vi "PLS Main.vi"(8 "error in (no error)":errorcluster, 9 "Aufnahme":bool caption="Record", 10 "Stop":bool, 11 "Play":bool) -> (0 "error out":errorcluster, 3 "Set Information":T1 {"Channels"."Intensität" min=0.0 max=100.0 step=1.0 format="%#.0f"})   [LabVIEW 2010]
doc: "User Interface für die Party Licht Steuerung"
uses:
  Controls/tlc_Cue_Information.ctl
  Controls/channel.ctl
  Controls/tlc_Consumer Control.ctl
  Controls/tlc_Functions.ctl
  Controls/tlc_User Interface Command.ctl
  Controls/tlc_User Interface Data Type.ctl
  Modules/Error/tlc_Error Module Command Control.ctl
  Modules/File/tlc_File_Command Control.ctl
  Modules/Cue/tlc_Cue_Information Command.ctl
  Integration/tlc_Record.vi
  Integration/tlc_Record Dialog Box.vi
panel:
  out "Cue List":i32(listbox)
  # "Ablaufkontrolle"
  # "Set Information"
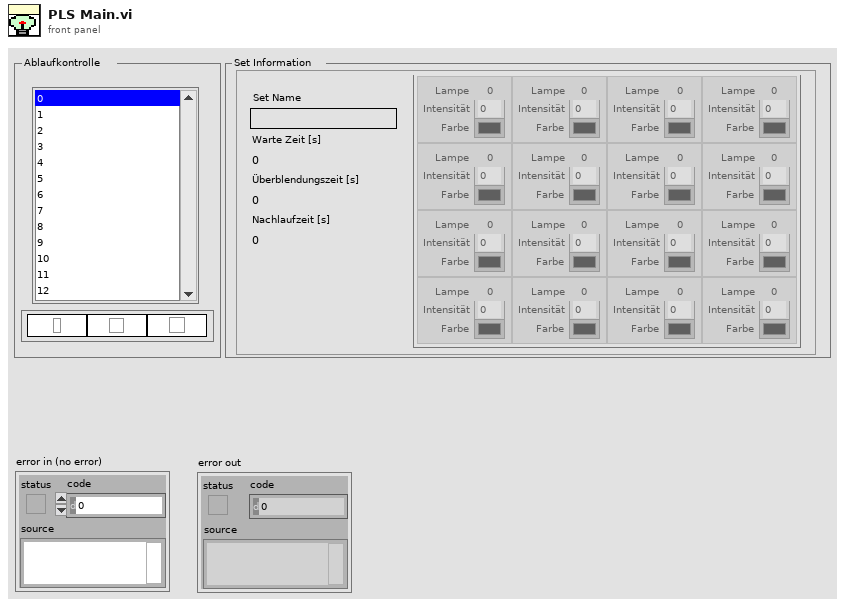
[diagram p1: front panel]
types:
  T1 = typedef "tlc_Cue_Information.ctl" = cluster{"Cue Name":string, "Wait Time (s)":u32, "Fade Time (s)":u32, "Follow Time (s)":u32, "Channels":T2[][]}
  T2 = typedef "channel.ctl" = cluster{"Intensität":dbl, " Farbe":u32, "Channel":i32}
  T3 = typedef "tlc_Error Module Command Control.ctl" = enum16{"Initialize", "Handle Errors", "Report Errors"}
  T4 = typedef "tlc_User Interface Command.ctl" = cluster{"Data Type":T5, "Data":variant}
  T5 = typedef "tlc_User Interface Data Type.ctl" = enum16{"Initialize", "Initialize Front Panel", "Update Front Panel Channels", "Select Cue in Cue List", "Enable/Disable Front Panel Controls", "Update Cue List", "Stop"}
  T6 = typedef "tlc_Consumer Control.ctl" = cluster{"Command":T7, "Data":variant}
  T7 = typedef "tlc_Functions.ctl" = enum16{"Initialize", "Record", "Load", "Save", "Play", "Stop", "Exit"}
  T8 = typedef "tlc_File_Command Control.ctl" = enum16{"Init", "Speicher Lichtersets", "Lade Lichtersets", "Ende"}
  T9 = typedef "tlc_Cue_Information Command.ctl" = enum16{"Add Lichtset", "Get Lichtset Werte", "Set Lichtset Werte", "Get Anzahl Lichtersets", "Init", "Get Leeres Lichterset"}
  T10 = enum32{"invalid app kind", "Development System", "Run Time System", "Student Edition", "Embedded LabVIEW", "Evaluation", "Custom"}
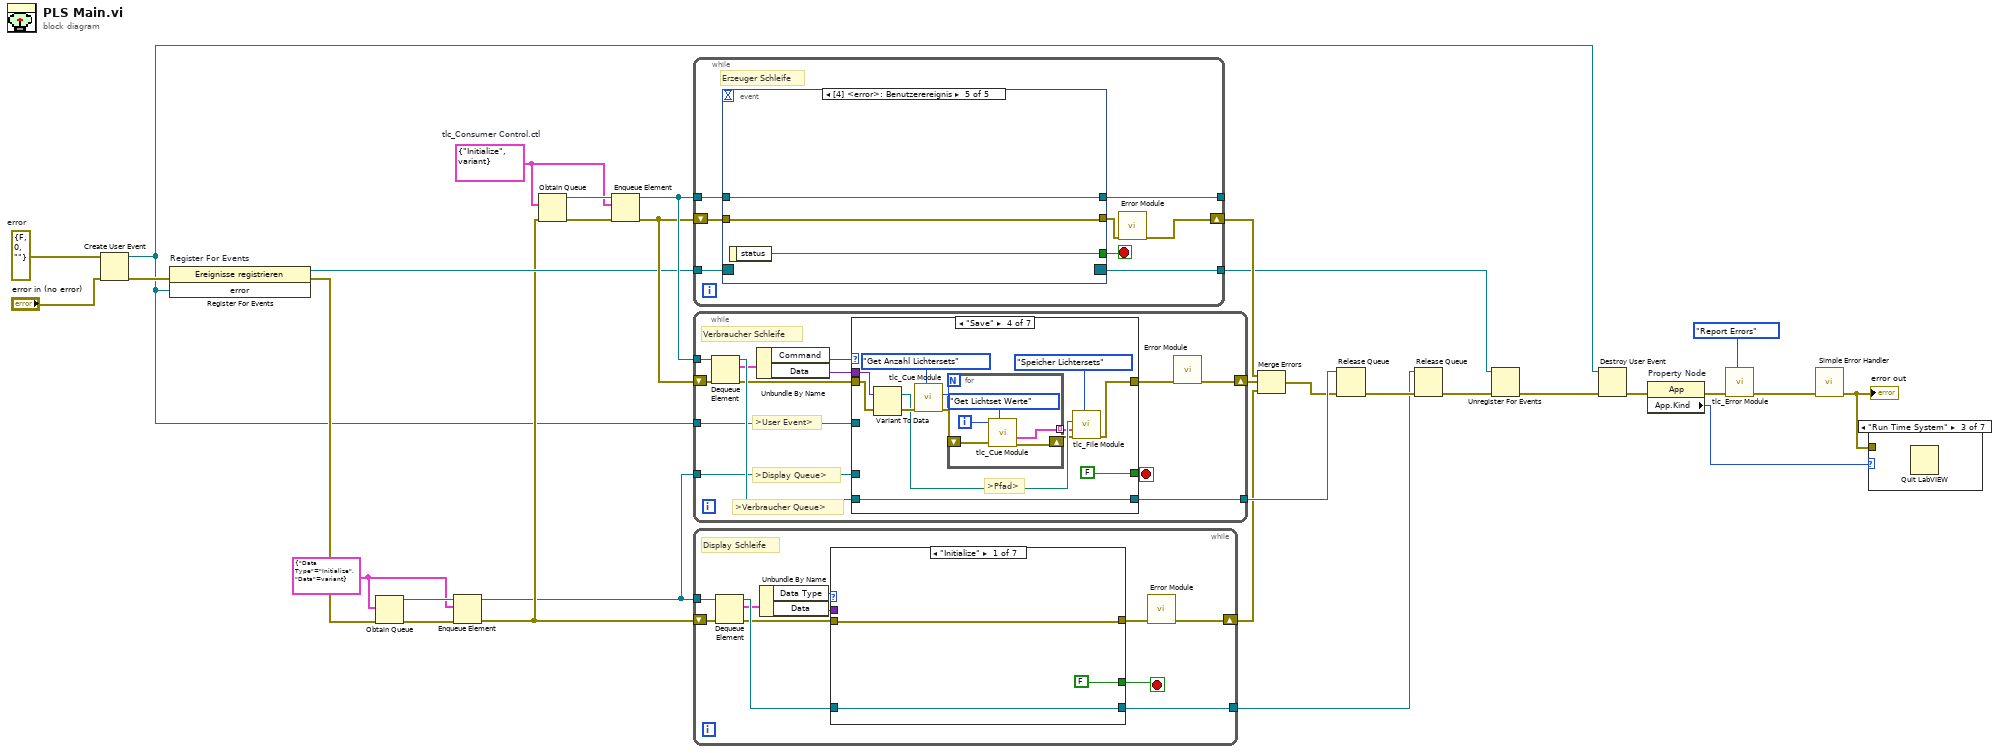
[diagram p0: block diagram]
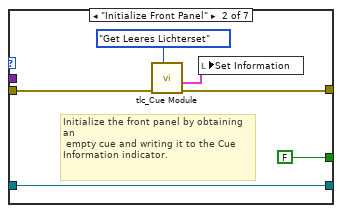
[diagram p8: hidden frame]
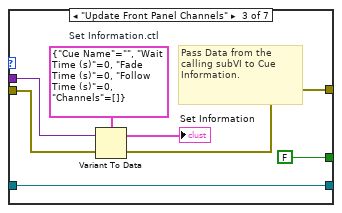
[diagram p9: hidden frame]
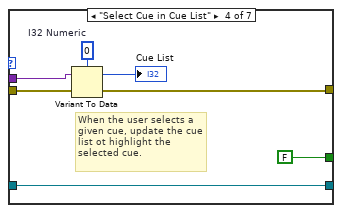
[diagram p10: hidden frame]
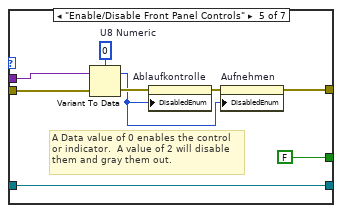
[diagram p11: hidden frame]
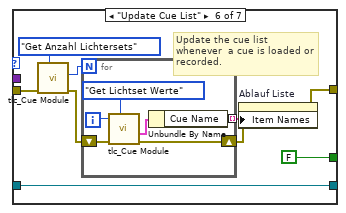
[diagram p12: hidden frame]
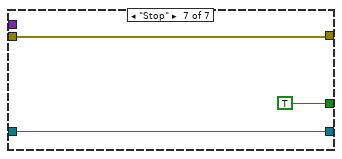
[diagram p13: hidden frame]
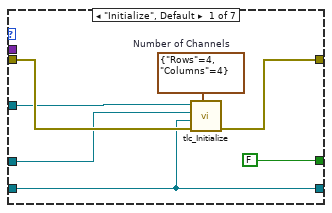
[diagram p14: hidden frame]
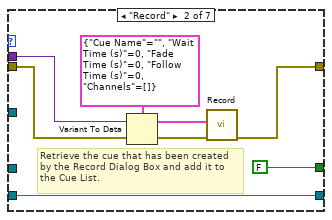
[diagram p15: hidden frame]
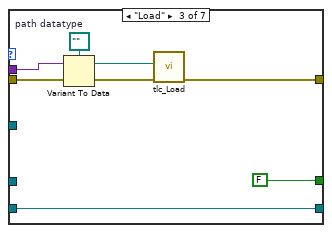
[diagram p16: hidden frame]
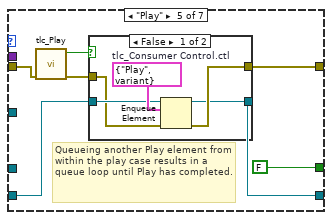
[diagram p17: hidden frame]
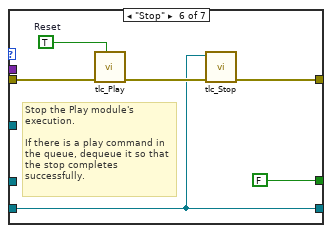
[diagram p19: hidden frame]
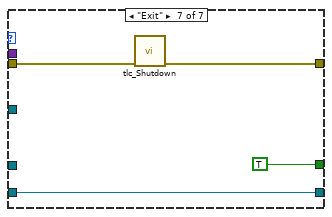
[diagram p20: hidden frame]
diagram:
  w15 = T4 {"Data Type"=enum."Initialize", "Data"=variant} ("tlc_User Interface Command.ctl")
  w27 = errorcluster {"status"=FALSE, "code"=0, "source"=""}  # error
  w29 = T6 {"Command"=enum."Initialize", "Data"=variant}  # tlc_Consumer Control.ctl
  n1 = Create User Event(user event datatype=w27, error in="error in (no error)") -> (user event=w9:refnum<user-event>, error out=w26:errorcluster)
  n2 = register-events "Register For Events"(error in=w26, w9) -> (reference out=w25:refnum<event-registration>, error out=w14:errorcluster)  [unwired: 1 in]
  n3 = Obtain Queue(element data type=w15, error in (no error)=w14) -> (queue out=w16:refnum<queue>, error out=w17:errorcluster)  [unwired: 3 in, 1 out]
  n4 = Enqueue Element(queue=w16, element=w15, error in (no error)=w17) -> (queue out=w8:refnum<queue>, error out=w13:errorcluster)  [unwired: 1 in, 1 out]
  n5 = Obtain Queue(element data type=w29, error in (no error)=w13) -> (queue out=w32:refnum<queue>, error out=w31:errorcluster)  [unwired: 3 in, 1 out]
  n6 = Enqueue Element(queue=w32, element=w29, error in (no error)=w31) -> (queue out=w30:refnum<queue>, error out=w28:errorcluster)  [unwired: 1 in, 1 out]
  n7 = while {
    shift-right: [w33] -> w23
    shift-left: w28 -> [w42]
    tunnel: w30 -> [w45]
    tunnel: [w43] -> w21
    tunnel: w9 -> [w37]
    tunnel: w8 -> [w36]
    stop <- w38 stop-if-true
    # ">Display Queue>"
    # ">Verbraucher Queue>"
    # ">User Event>"
    # "Verbraucher Schleife"
    n8 = Dequeue Element(queue=w45, error in (no error)=w42) -> (queue out=w44:refnum<queue>, element=w41:T6, error out=w39:errorcluster)  [unwired: 1 in, 1 out]
    n9 = Unbundle By Name(w41) -> ("Command"=w40:T7, "Data"=w35:variant)
    n10 = case shown="\"Save\"" w40 {
      tunnel: w44 -> [w48 w60 w68 w81 w89 w101 w110]
      tunnel: [w48 w60 w68 w81 w87 w101 w110] -> w43
      tunnel: w39 -> [w50 w53 w65 w78 w92 w104 w108]
      tunnel: [w49 w57 w62 w70 w88 w103 w107] -> w34
      tunnel: [FALSE FALSE FALSE FALSE FALSE FALSE TRUE] -> w38
      tunnel: w35 -> [_ w54 w66 w79 _ _ _]
      tunnel: w37 -> [w47 _ _ _ _ _ _]
      tunnel: w36 -> [w46 _ _ _ _ _ _]
      frame "Initialize", Default {
        w51 = cluster{"Rows":i32, "Columns":i32} {"Rows"=4, "Columns"=4}  # Number of Channels
        n11 = call "tlc_Initialize.vi"("Anzahl Kanäle"=w51, "error in (no error)"=w50, "Consumer Queue Reference.ctl"=w48, "Display Queue Reference.ctl"=w46, "User Event Reference.ctl"=w47) -> ("error out"=w49:errorcluster)  [unwired: 6 in]
      }
      frame "Record" {
        # "Retrieve the cue that has been created by the Record Dialog Box and add it to the Cue List."
        n12 = Variant To Data(error in=w53, Variant=w54, type=T1 {"Cue Name"="", "Wait Time (s)"=0, "Fade Time (s)"=0, "Follow Time (s)"=0, "Channels"=[]} ("tlc_Cue_Information.ctl")) -> (error out=w58:errorcluster, data=w56:T1)
        n13 = call "Record.vi"("error in (no error)"=w58, "Cue"=w56) -> ("error out"=w57:errorcluster)  [unwired: 9 in]
      }
      frame "Load" {
        w61 = path ""  # path datatype
        n14 = Variant To Data(error in=w65, Variant=w66, type=w61) -> (error out=w64:errorcluster, data=w63:path)
        n15 = call "tlc_Load.vi"("error in (no error)"=w64, "Path"=w63) -> ("error out"=w62:errorcluster)  [unwired: 9 in]
      }
      frame "Save" {
        # ">Pfad>"
        n16 = Variant To Data(error in=w78, Variant=w79) -> (error out=w77:errorcluster, data=w75:path)  [unwired: 1 in]
        n17 = call "tlc_Cue Module.vi"("Command"=tlc_Cue_Information_Command."Get Anzahl Lichtersets", "error in (no error)"=w77) -> ("error out"=w73:errorcluster, "Number of Cues"=w74:i32)  [unwired: 6 in, 1 out]
        n18 = for {
          N: w74 -> [_]
          shift-right: [w85] -> w72
          shift-left: w73 -> [w86]
          tunnel: [w84] -> w71 mode=indexing
          i -> [w83]
          n19 = call "tlc_Cue Module.vi"("Command"=tlc_Cue_Information_Command."Get Lichtset Werte", "error in (no error)"=w86, "Cue Index"=w83) -> ("error out"=w85:errorcluster, "Cue Output"=w84:T1)  [unwired: 5 in, 1 out]
        }
        n20 = call "tlc_File Module.vi"("Command"=tlc_File_Command_Control."Speicher Lichtersets", "error in (no error)"=w72, "1D Array Input aus Lichtersets"=w71, "Pfad"=w75) -> ("error out"=w70:errorcluster)  [unwired: 6 in, 1 out]
      }
      frame "Play" {
        # "Queueing another Play element from within the play case results in a queue loop until Play has completed."
        n21 = call "tlc_Play.vi"("error in (no error)"=w92) -> ("error out"=w90:errorcluster, "Stop?"=w91:bool)  [unwired: 9 in]
        n22 = case shown="False" w91 {
          tunnel: w90 -> [w95 w100]
          tunnel: w89 -> [w97 w99]
          tunnel: [w96 w100] -> w88
          tunnel: [w94 w99] -> w87
          frame False {
            w98 = T6 {"Command"=enum."Play", "Data"=variant}  # tlc_Consumer Control.ctl
            n23 = Enqueue Element(queue=w97, element=w98, error in (no error)=w95) -> (queue out=w94:refnum<queue>, error out=w96:errorcluster)  [unwired: 1 in, 1 out]
          }
          frame True {
          }
        }
      }
      frame "Stop" {
        w102 = TRUE  # Reset
        # "Stop the Play module's execution.\n\nIf there is a play command in the queue, dequeue it so that the stop completes successfully."
        n24 = call "tlc_Play.vi"("Reset"=w102, "error in (no error)"=w104) -> ("error out"=w105:errorcluster)  [unwired: 8 in, 1 out]
        n25 = call "tlc_Stop.vi"("error in"=w105, "tlc_Consumer Queue Reference.ctl"=w101) -> ("error out"=w103:errorcluster)  [unwired: 9 in]
      }
      frame "Exit" {
        n26 = call "tlc_Shutdown.vi"("error in (no error)"=w108) -> ("error out"=w107:errorcluster)  [unwired: 10 in]
      }
    }
    n27 = call "Error Module.vi"("error in (no error)"=w34) -> ("error out"=w33:errorcluster)  [unwired: 9 in, 1 out]
  }
  n28 = while {
    shift-right: [w111] -> w7
    shift-left: w13 -> [w119]
    tunnel: [w120] -> w10
    tunnel: w8 -> [w114]
    stop <- w116 stop-if-true
    # "Display Schleife"
    n29 = Dequeue Element(queue=w114, error in (no error)=w119) -> (queue out=w121:refnum<queue>, element=w118:T4, error out=w117:errorcluster)  [unwired: 1 in, 1 out]
    n30 = Unbundle By Name(w118) -> ("Data Type"=w113:T5, "Data"=w115:variant)
    n31 = case shown="\"Initialize\"" w113 {
      tunnel: w121 -> [w123 w130 w137 w144 w153 w162 w170]
      tunnel: [w123 w130 w137 w144 w153 w162 w170] -> w120
      tunnel: w117 -> [w124 w127 w135 w142 w151 w160 w171]
      tunnel: [w124 w126 w133 w140 w146 w158 w171] -> w112
      tunnel: [FALSE FALSE FALSE FALSE FALSE FALSE TRUE] -> w116
      tunnel: w115 -> [_ _ w134 w141 w150 _ _]
      frame "Initialize" {
      }
      frame "Initialize Front Panel" {
        # "Initialize the front panel by obtaining an\n empty cue and writing it to the Cue Information indicator."
        n32 = call "tlc_Cue Module.vi"("Command"=tlc_Cue_Information_Command."Get Leeres Lichterset", "error in (no error)"=w127) -> ("error out"=w126:errorcluster, "Cue Output"=w125:T1)  [unwired: 6 in, 1 out]
        n33 = local write "Set Information"(w125) -> ()
      }
      frame "Update Front Panel Channels" {
        w131 = T1 {"Cue Name"="", "Wait Time (s)"=0, "Fade Time (s)"=0, "Follow Time (s)"=0, "Channels"=[]}  # Set Information.ctl
        # "Pass Data from the calling subVI to Cue Information."
        n34 = Variant To Data(error in=w135, Variant=w134, type=w131) -> (error out=w133:errorcluster, data=→"Set Information":T1)
      }
      frame "Select Cue in Cue List" {
        w138 = 0  # I32 Numeric
        # "When the user selects a given cue, update the cue list ot highlight the selected cue."
        n35 = Variant To Data(error in=w142, Variant=w141, type=w138) -> (error out=w140:errorcluster, data=→"Cue List":i32)
      }
      frame "Enable/Disable Front Panel Controls" {
        w149 = 0  # U8 Numeric
        # "A Data value of 0 enables the control or indicator.  A value of 2 will disable them and gray them out."
        n36 = Variant To Data(error in=w151, Variant=w150, type=w149) -> (error out=w148:errorcluster, data=w145:i32)
        n37 = property on="Ablaufkontrolle" class="Listenfeld (strikt)"(error in=w148, "DisabledEnum"=w145) -> (error out=w147:errorcluster)  [unwired: 1 in, 1 out]
        n38 = property on="Aufnehmen" class="Bool."(error in=w147, "DisabledEnum"=w145) -> (error out=w146:errorcluster)  [unwired: 1 in, 1 out]
      }
      frame "Update Cue List" {
        # "Update the cue list whenever  a cue is loaded or recorded."
        n39 = call "tlc_Cue Module.vi"("Command"=tlc_Cue_Information_Command."Get Anzahl Lichtersets", "error in (no error)"=w160) -> ("error out"=w155:errorcluster, "Number of Cues"=w157:i32)  [unwired: 6 in, 1 out]
        n40 = for {
          N: w157 -> [_]
          tunnel: [w165] -> w156 mode=indexing
          shift-right: [w164] -> w154
          shift-left: w155 -> [w163]
          i -> [w167]
          n41 = call "tlc_Cue Module.vi"("Command"=tlc_Cue_Information_Command."Get Lichtset Werte", "error in (no error)"=w163, "Cue Index"=w167) -> ("error out"=w164:errorcluster, "Cue Output"=w166:T1)  [unwired: 5 in, 1 out]
          n42 = Unbundle By Name(w166) -> ("Cue Name"=w165:string)
        }
        n43 = property on="Ablauf Liste" class="Listenfeld (strikt)"(error in=w154, "Item Names"=w156) -> (error out=w158:errorcluster)  [unwired: 1 in, 1 out]
      }
      frame "Stop" {
      }
    }
    n44 = call "Error Module.vi"("error in (no error)"=w112) -> ("error out"=w111:errorcluster)  [unwired: 9 in, 1 out]
  }
  n45 = while {
    shift-right: [w172] -> w22
    shift-left: w28 -> [w178]
    tunnel: w25 -> [w175]
    tunnel: [w174] -> w19
    tunnel: w30 -> [w179]
    tunnel: [w176] -> _
    stop <- w177 stop-if-true
    # "Erzeuger Schleife"
    n46 = event shown="[4] <error>: Benutzerereignis" {
      selector: w175 -> [_ _ _ _ _]
      dyn-events: [_ _ _ _ _] -> w174
      timeout: _ -> [_ _ _ _ _]
      tunnel: w179 -> [w186 w194 w215 w221 w282]
      tunnel: w178 -> [w185 w191 w208 w220 w281]
      tunnel: [w184 w193 w214 w218 w281] -> w173
      tunnel: [FALSE FALSE FALSE w217 w283] -> w177
      tunnel: [w180 w192 w210 w219 w282] -> w176
      event "Play": Value Change {
        w183 = T6 {"Command"=enum."Initialize", "Data"=variant}  # tlc_Consumer Control.ctl
        n47 = event-data() -> ()  [unwired: 1 in, 1 out]
        n48 = Bundle By Name(cluster=w183, "Command"=tlc_Functions."Play") -> (w182:T6)
        n49 = Enqueue Element(queue=w186, element=w182, error in (no error)=w185) -> (queue out=w180:refnum<queue>, error out=w184:errorcluster)  [unwired: 1 in, 1 out]
      }
      event "Aufnahme": Value Change {
        # "Obtain a queue from the user and send the cue to the consumer loop."
        n50 = event-data() -> ()  [unwired: 1 in, 1 out]
        n51 = call "Record Dialog Box.vi"("error in (no error)"=w191) -> ("error out"=w190:errorcluster, "Output Cue"=w188:T1, "Cancelled?"=w189:bool)  [unwired: 8 in]
        n52 = case shown="False" w189 {
          tunnel: w194 -> [w204 w206]
          tunnel: w190 -> [w203 w205]
          tunnel: [w202 w205] -> w193
          tunnel: [w198 w206] -> w192
          tunnel: w188 -> [w196 _]
          frame False {
            n53 = To Variant(anything=w196) -> (Variant=w197:variant)
            n54 = Bundle By Name(cluster=T6 {"Command"=enum."Initialize", "Data"=variant} ("tlc_Consumer Control.ctl"), "Command"=tlc_Functions."Record", "Data"=w197) -> (w200:T6)
            n55 = Enqueue Element(queue=w204, element=w200, error in (no error)=w203) -> (queue out=w198:refnum<queue>, error out=w202:errorcluster)  [unwired: 1 in, 1 out]
          }
          frame True {
          }
        }
      }
      event "Stop": Value Change {
        # "Clear the consumer loop queue, then stop the consumer loop."
        n56 = event-data() -> ()  [unwired: 1 in, 1 out]
        n57 = Flush Queue(queue=w215, error in (no error)=w208) -> (queue out=w209:refnum<queue>, error out=w207:errorcluster)  [unwired: 1 out]
        n58 = Bundle By Name(cluster=T6 {"Command"=enum."Initialize", "Data"=variant} ("tlc_Consumer Control.ctl"), "Command"=tlc_Functions."Stop") -> (w212:T6)
        n59 = Enqueue Element "Element einfügen"(queue=w209, element=w212, error in (no error)=w207) -> (queue out=w210:refnum<queue>, error out=w214:errorcluster)  [unwired: 1 in, 1 out]
      }
      event Menu Selection (User) {
        n60 = event-data() -> ("ItemTag"=w222:string)  [unwired: 1 in]
        n61 = case shown="\"Save\"" w222 {
          tunnel: w221 -> [w223 w245 w277 w280]
          tunnel: w220 -> [w231 w253 w275 w279]
          tunnel: [w227 w249 w276 w280] -> w219
          tunnel: [w228 w250 w274 w279] -> w218
          tunnel: [FALSE FALSE TRUE FALSE] -> w217
          frame "Save" {
            n62 = call "File Dialog"("error in"=w231) -> ("selected path"=w224:path, "exists"=w230:bool, "cancelled"=w229:bool, "error out"=w226:errorcluster)  [unwired: 11 in]
            n63 = Compound Arithmetic op=OR(w230, invert w229) -> (w225:bool)
            n64 = case shown="True" w225 {
              tunnel: [w235 w244] -> w228
              tunnel: [w233 w243] -> w227
              tunnel: w226 -> [w236 w242]
              tunnel: w224 -> [_ w241]
              tunnel: w223 -> [w233 w237]
              frame False {
                n65 = call "Clear Specific Error.vi"("error in (no error)"=w236, "Code"=43) -> ("error out"=w235:errorcluster)  [unwired: 5 in]
              }
              frame True {
                n66 = To Variant(anything=w241) -> (Variant=w239:variant)
                n67 = Bundle By Name(cluster=T6 {"Command"=enum."Save", "Data"=variant} ("tlc_Consumer Control.ctl"), "Data"=w239) -> (w238:T6)
                n68 = Enqueue Element(queue=w237, element=w238, error in (no error)=w242) -> (queue out=w243:refnum<queue>, error out=w244:errorcluster)  [unwired: 1 in, 1 out]
              }
            }
          }
          frame "Open" {
            n69 = call "File Dialog2"("error in"=w253) -> ("selected path"=w246:path, "exists"=w252:bool, "cancelled"=w251:bool, "error out"=w248:errorcluster)  [unwired: 11 in]
            n70 = Compound Arithmetic op=OR(w252, invert w251) -> (w247:bool)
            n71 = case shown="True" w247 {
              tunnel: [w256 w269] -> w250
              tunnel: [w255 w268] -> w249
              tunnel: w248 -> [w257 w267]
              tunnel: w246 -> [_ w266]
              tunnel: w245 -> [w255 w262]
              frame False {
                n72 = disable-structure shown="Aktiviert" {
                  disable-tunnel: w257 -> [w260 w261]
                  disable-tunnel: [w259 w261] -> w256
                  frame Enabled {
                    n73 = call "Clear Specific Error.vi"("error in (no error)"=w260, "Code"=43) -> ("error out"=w259:errorcluster)  [unwired: 5 in]
                  }
                  frame Disabled {
                  }
                }
              }
              frame True {
                w265 = T6 {"Command"=enum."Load", "Data"=variant}  # tlc_Consumer Control.ctl
                n74 = To Variant(anything=w266) -> (Variant=w264:variant)
                n75 = Bundle By Name(cluster=w265, "Data"=w264) -> (w263:T6)
                n76 = Enqueue Element(queue=w262, element=w263, error in (no error)=w267) -> (queue out=w268:refnum<queue>, error out=w269:errorcluster)  [unwired: 1 in, 1 out]
              }
            }
          }
          frame "Exit" {
            w273 = T6 {"Command"=enum."Initialize", "Data"=variant}  # tlc_Consumer Control.ctl
            n77 = Bundle By Name(cluster=w273, "Command"=tlc_Functions."Exit") -> (w270:T6)
            n78 = Enqueue Element(queue=w277, element=w270, error in (no error)=w275) -> (queue out=w276:refnum<queue>, error out=w274:errorcluster)  [unwired: 1 in, 1 out]
          }
          frame Default {
          }
        }
      }
      event User Event {
        n79 = event-data() -> ("status"=w283:bool)  [unwired: 1 in]
      }
    }
    n80 = call "Error Module.vi"("error in (no error)"=w173) -> ("error out"=w172:errorcluster)  [unwired: 9 in, 1 out]
  }
  n81 = Merge Errors(w22, w23, w7) -> (w20:errorcluster)
  n82 = Release Queue(queue=w21, error in (no error)=w20) -> (error out=w12:errorcluster)  [unwired: 1 in, 2 out]
  n83 = Release Queue(queue=w10, error in (no error)=w12) -> (error out=w11:errorcluster)  [unwired: 1 in, 2 out]
  n84 = Unregister For Events(event registration refnum=w19, error in=w11) -> (error out=w18:errorcluster)
  n85 = Destroy User Event(user event=w9, error in=w18) -> (error out=w4:errorcluster)
  n86 = property on="Property Node" class="App"(error in=w4) -> (error out=w3:errorcluster, "App.Kind"=w2:T10)  [unwired: 1 in, 1 out]
  n87 = call "tlc_Error Module.vi"("Command (Handle Errors)"=tlc_Error_Module_Command_Control."Report Errors" ("Command (Handle Errors"), "error in (no error)"=w3) -> ("error out"=w5:errorcluster)  [unwired: 8 in, 1 out]
  n88 = call <vilib>:"Simple Error Handler.vi"("error in (no error)"=w5) -> ("error out"=w1:errorcluster)  [unwired: 4 in, 4 out]
  "error out" <- w1
  n89 = case shown="\"Run Time System\"" w2 {
    tunnel: w1 -> [_ _ _ _ _ _ _]
    frame "invalid app kind", Default {
    }
    frame "Development System" {
    }
    frame "Run Time System" {
      n90 = Quit LabVIEW() -> ()  [unwired: 1 in]
    }
    frame "Student Edition" {
    }
    frame "Embedded LabVIEW" {
    }
    frame "Evaluation" {
    }
    frame "Custom" {
    }
  }
